vi "Display Loader.vi"(8 "error in (no error)":errorcluster, 10 "VI in":refnum<vi>, 11 "application ref in":refnum<vi>) -> (0 "error out":errorcluster, 3 "application ref out":refnum<vi>)   [LabVIEW 2019, in "gRPC Scripting Tools.lvlib"]
uses:
  gRPC Scripting Tools.lvlib
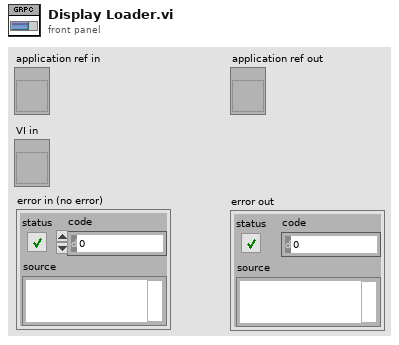
[diagram p1: front panel]
types:
  T1 = enum16{"Always On", "Always Off", "Off While Running"}
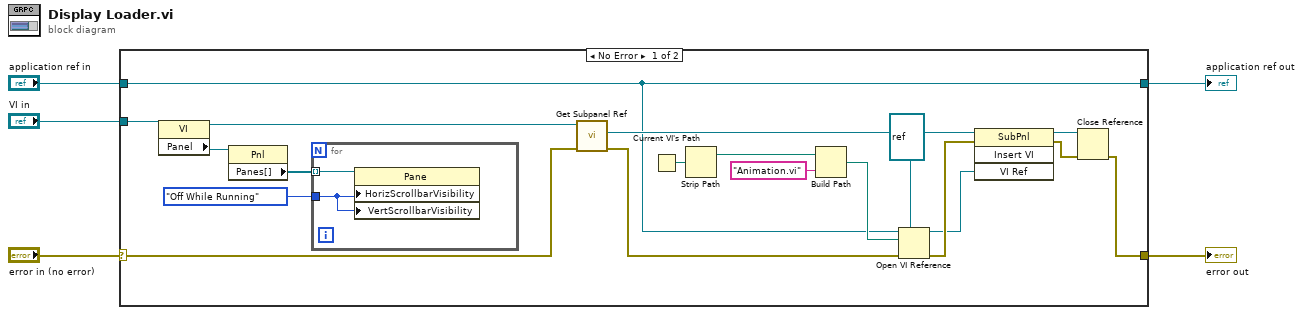
[diagram p0: block diagram]
diagram:
  n1 = case shown="No Error" "error in (no error)" {
    selector: "error in (no error)" -> [w16 w28]
    tunnel: [w12 w28] -> w5
    tunnel: "VI in" -> [w10 _]
    tunnel: "application ref in" -> [w11 w27]
    tunnel: [w11 w27] -> w1
    frame No Error {
      n2 = property class="VI"(reference=w10) -> (reference out=w6:refnum<vi>, "Panel"=w9:refnum<vi>)  [unwired: 1 in, 1 out]
      n3 = property class="Pnl"(reference=w9) -> ("Panes[]"=w8:refnum<vi>[])  [unwired: 1 in, 2 out]
      n4 = for {
        tunnel: w8 -> [w26] mode=indexing
        tunnel: T1."Off While Running" ("Horizontal Scrollbar Visibility") -> [w25]
        n5 = property class="Pane"(reference=w26, "HorizScrollbarVisibility"=w25, "VertScrollbarVisibility"=w25) -> ()  [unwired: 1 in, 2 out]
      }
      n6 = call "Get Subpanel Ref.vi"("error in (no error)"=w16, "Owner VI in"=w6) -> ("error out"=w15:errorcluster, "SubPanel out"=w24:refnum<vi>)  [unwired: 8 in]
      n7 = Current VI's Path() -> (path=w21:path)
      n8 = Strip Path(path=w21) -> (stripped path=w22:path)  [unwired: 1 out]
      n9 = Build Path(base path=w22, name or relative path="Animation.vi") -> (appended path=w14:path)
      n10 = Open VI Reference(type specifier VI Refnum (for type only)=refnum<vi> refnum, application reference (local)=w11, vi path=w14, error in (no error)=w15) -> (vi reference=w13:refnum<vi>, error out=w20:errorcluster)  [unwired: 2 in]
      n11 = invoke class="SubPnl" method="Insert VI"(reference=w24, error in=w20, "VI Ref"=w13) -> (reference out=w18:refnum<vi>, error out=w19:errorcluster)  [unwired: 1 in, 2 out]
      n12 = Close Reference(reference=w18, error in (no error)=w19) -> (error out=w12:errorcluster)
    }
    frame Error {
    }
  }
  "error out" <- w5
  "application ref out" <- w1
